vi "show_sensitivity.vi"() -> ()   [LabVIEW 2014]
panel:
  in  "show sensitivity (ana denge  y)":dbl
  in  "show sensitivity (ana denge  x)":dbl
  in  "show sensitivity (kelvin  y)":dbl
  in  "show sensitivity (kelvin  x)":dbl
  in  "show sensitivity (1R  y)":dbl
  in  "show sensitivity (1R  x)":dbl
  in  "show sensitivity (10R  y)":dbl
  in  "show sensitivity (10R  x)":dbl
  in  "show sensitivity (wagner  y)":dbl
  in  "show sensitivity (wagner  x)":dbl
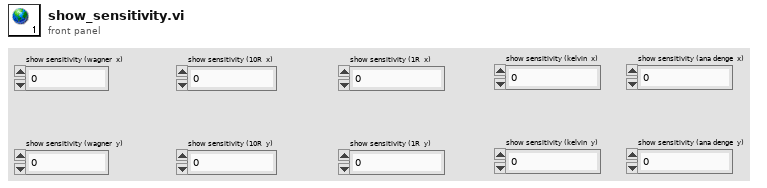
[diagram p1: front panel]
diagram:
